vi "create Map.vi"(8 "error in (no error)":errorcluster, 10 "Board":refnum<class "Board.lvclass">, 11 "Map in":refnum<class "Map.lvclass">) -> (0 "error out":errorcluster, 3 "Map out":refnum<class "Map.lvclass">)   [LabVIEW 2019, in "Map.lvclass"]
uses:
  Map.lvclass
  Board/Board.lvclass
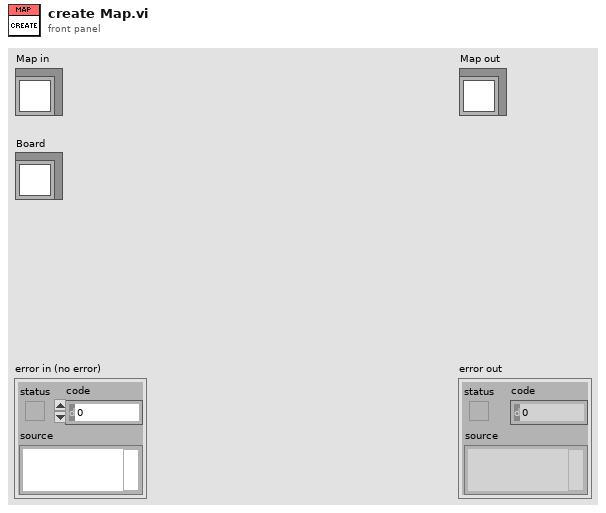
[diagram p1: front panel]
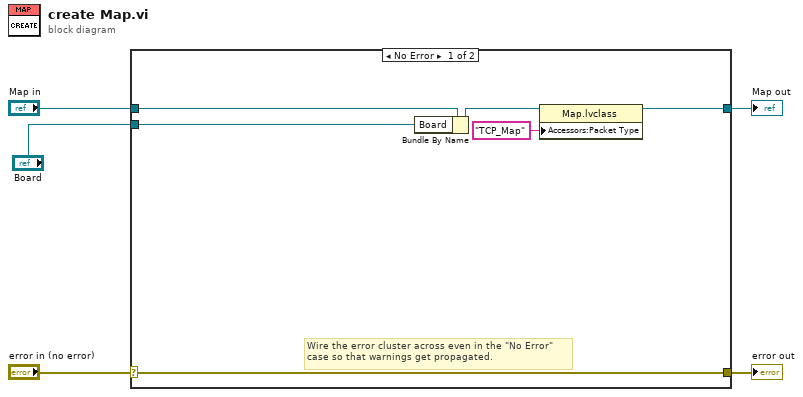
[diagram p0: block diagram]
diagram:
  n1 = case shown="No Error" "error in (no error)" {
    selector: "error in (no error)" -> [w10 w13]
    tunnel: [w10 w13] -> w4
    tunnel: [w7 w12] -> w2
    tunnel: "Map in" -> [w11 w12]
    tunnel: "Board" -> [w8 _]
    frame No Error {
      # "Wire the error cluster across even in the \"No Error\"\ncase so that warnings get propagated."
      n2 = Bundle By Name(cluster=w11, "Board"=w8) -> (w9:refnum<class "Map.lvclass">)
      n3 = property class="Map.lvclass"(reference=w9, "Accessors:Packet Type"="TCP_Map" ("Packet Type")) -> (reference out=w7:refnum<class "Map.lvclass">)  [unwired: 1 in, 1 out]
    }
    frame Error {
    }
  }
  "error out" <- w4
  "Map out" <- w2
